vi "SwitchIconByNumber.vi"(7 "Index":i32, 8 "error in (no error)":errorcluster, 10 "Icon Array Ref":refnum<vi>, 11 "Switch Values ref":refnum<vi>) -> (0 "error out":errorcluster, 1 "Val out":bool, 2 "Icon Array ref out":refnum<vi>, 3 "Switch Values ref out":refnum<vi>)   [LabVIEW 2023]
doc: "This VI switches both Icons (negate image) and Icons Values at specified index. \n\nSwitch Values ref - a reference to the array of booleans. \nIcon Array ref - a reference to the Icons image array.\nIndex - a value of the index to switch. \n\nSwitch Values ref out - Booleans array reference out. \nIcons Array ref out - Icons array reference out. \nVal out - The new value that was set."
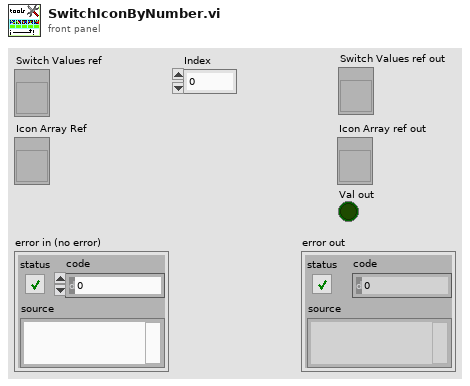
[diagram p1: front panel]
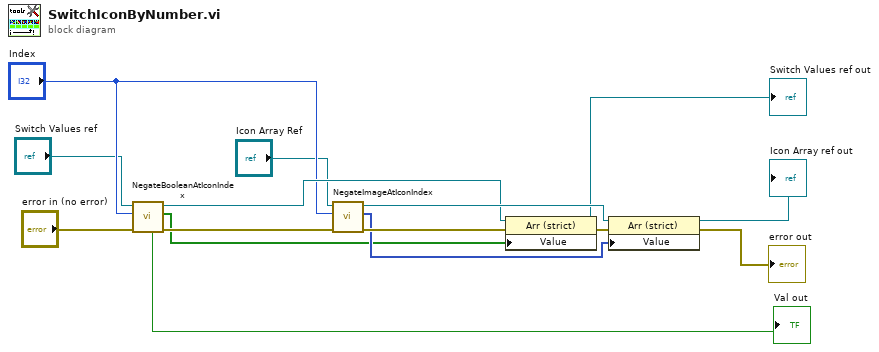
[diagram p0: block diagram]
diagram:
  n1 = call "NegateBooleanAtIconIndex.vi"("error in (no error)"="error in (no error)", "Index"="Index", "Boolean Array ref  in"="Switch Values ref") -> ("error out"=w11:errorcluster, "New Value"=w4:bool[], "Boolean Array Ref Out"=w9:refnum<vi>, "Val out"=→"Val out":bool)  [unwired: 4 in, 1 out]
  n2 = call "NegateImageAtIconIndex.vi"("error in (no error)"=w11, "Index"="Index", "Image Array ref in"="Icon Array Ref") -> ("error out"=w12:errorcluster, "New Image Array Value"=w5:picture[], "Array ref out"=w10:refnum<vi>)  [unwired: 5 in, 1 out]
  n3 = property on="Property Node" class="Arr (strict)"(reference=w9, error in=w12, "Value"=w4) -> (reference out=→"Switch Values ref out":refnum<vi>, error out=w13:errorcluster)
  n4 = property on="Property Node" class="Arr (strict)"(reference=w10, error in=w13, "Value"=w5) -> (reference out=→"Icon Array ref out":refnum<vi>, error out=→"error out":errorcluster)
